vi "Main.vi"(11 "Module Admin":refnum<class "Delacor_lib_QMH_Cloneable Module Admin.lvclass">) -> ()   [LabVIEW 2024, in "Clon.lvlib"]
doc: "This template is based off of the Queued Message Handler design pattern and the Queued Message Handler project template that ships with LabVIEW.\n\nThe main difference is that the queue is private to this module and communication between modules is performed via Broadcast and Request events.\n\nRequest events are wrapped in public API methods and are handled in the Event Handling Loop (EHL) of this VI. Any module can register for Broadcast events sent by this module. The EHL generates messages based on user interface actions.\n\nThe Message Handling Loop (MHL) processes messages generated by the EHL, or by other messages. The messages are string values, so new messages can be added easily to the Message Cases case structure in the MHL. Each message cluster can also provide an optional value for Message Data, which is a variant that can be converted to whatever message-specific data is required.\n_____\nBased on DQMH Dev Tools: Project Template 7.1.0.1503."
uses:
  Clon.lvlib
  <vilib>/Delacor/Delacor QMH/Libraries/Cloneable Module Admin_class/Delacor_lib_QMH_Cloneable Module Admin.lvclass
  C:/Program Files (x86)/National Instruments/LabVIEW 2024/vi.lib/Delacor/Delacor QMH/Libraries/Module Admin_class/Delacor_lib_QMH_Module Admin.lvclass
  Module Data--cluster.ctl
  Do Something Argument--cluster.ctl
  <vilib>/Delacor/Delacor QMH/Libraries/Cloneable Module Admin_class/Delacor_lib_QMH_Cloneable Module Admin.lvclass/Delacor_lib_QMH_Cloneable Module Admin.ctl
  <vilib>/Delacor/Delacor QMH/Libraries/Message Queue_class/Delacor_lib_QMH_Message Queue.lvclass/Delacor_lib_QMH_Message Queue.ctl
  Do Something Else Argument--cluster.ctl
  Do Something Else and Wait for Reply Argument--cluster.ctl
  Do Something Else and Wait (Reply Payload)--cluster.ctl
  Stop Argument--cluster.ctl
  <vilib>/Delacor/Delacor QMH/Libraries/Module Admin_class/Delacor_lib_QMH_Module Admin.lvclass/Delacor_lib_QMH_Module Admin.ctl
  <vilib>/Utility/miscctls.llb/LVPointTypeDef.ctl
  <vilib>/Delacor/Delacor QMH/Libraries/Message Queue_class/Delacor_lib_QMH_Enqueue Message (Single).vi
  <vilib>/Delacor/Delacor QMH/Libraries/Cloneable Module Admin_class/Delacor_lib_QMH_Get Module ID.vi
  <vilib>/Delacor/Delacor QMH/Libraries/Module Admin_class/Delacor_lib_QMH_Get External Launch.vi
  <vilib>/Delacor/Delacor QMH/Libraries/Message Queue_class/Delacor_lib_QMH_Message Queue.lvclass
  Evento DEmo Argument--cluster.ctl
panel:
  out "error out":errorcluster
  out "X":dbl
  out "Status":string
  in  "Simulate EHL Error":bool
  in  "Simulate MHL Error":bool
  in  "Do Something Else <Replace Me>":bool
  in  "Do Something <Replace Me>":bool
  # "These controls have associated \"Value Changed\" events configured in the Event Structure on the diagram.\n\nReplace them (and reconfigure the Event Structure) with the controls you need for your application. \n\nOther processes communicate with this Module via its Public API (wrappers for its Request Events).\n\nThis Module communicates with other processes via its Broadcast Events.\nAny process that wants to receive these messages can register for this module's Broadcast events."
  # "This template is for the DQMH framework. See the block diagram for more information on how to use this template."
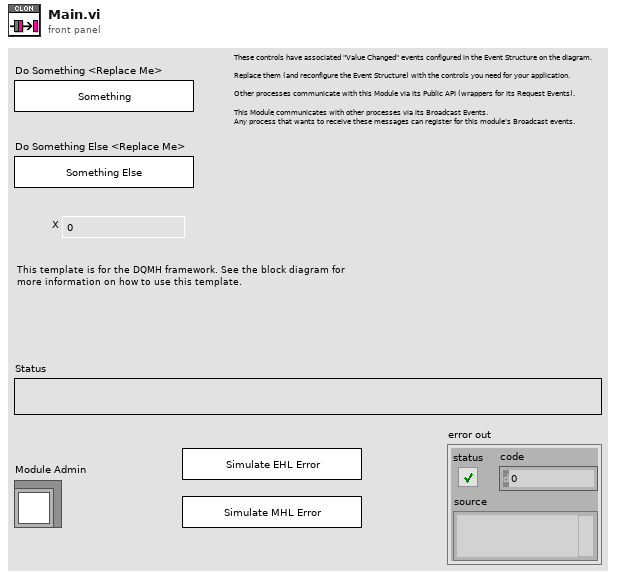
[diagram p1: front panel]
types:
  T1 = typedef "Clon.lvlib/Request Events--cluster.ctl" = cluster{"Stop Module":refnum<user-event>, "Do Something":refnum<user-event>, "Do Something Else":refnum<user-event>, "Do Something Else and Wait for Reply":refnum<user-event>, "Show Panel":refnum<user-event>, "Hide Panel":refnum<user-event>, "Show Diagram":refnum<user-event>, "Get Module Execution Status":refnum<user-event>, "Evento DEmo":refnum<user-event>}
  T2 = typedef "Clon.lvlib/Module Data--cluster.ctl" = cluster{"Status":string}
  T3 = typedef "Clon.lvlib/Do Something Argument--cluster.ctl" = cluster{"Module ID":i32, "Do Something Msg":string}
  T4 = typedef "Clon.lvlib/Do Something Else Argument--cluster.ctl" = cluster{"Module ID":i32, "Do Something Else Msg":string, "X":dbl}
  T5 = typedef "Clon.lvlib/Do Something Else and Wait for Reply Argument--cluster.ctl" = cluster{"Module ID":i32, "Do Something Else Msg":string, "X":dbl, "Wait Notifier":refnum<notifier>, "wait for reply":bool}
  T6 = enum32{"invalid lock state", "Not Locked", "Locked (No Password)", "Password-protected"}
  T7 = typedef "Clon.lvlib/Stop Argument--cluster.ctl" = cluster{"Module ID":i32, "Origin":string, "Exit via Stop Module Req?":bool, "Wait for Module to stop?":bool}
  T8 = typedef "Clon.lvlib/Evento DEmo Argument--cluster.ctl" = cluster{"Module ID":i32, "Numeric":dbl}
  T9 = typedef "LVPointTypeDef.ctl" = cluster{"Horizontal":i16, "Vertical":i16}
  T10 = enum32{"Invalid", "Standard", "Closed", "Hidden", "Minimized", "Maximized"}
  T11 = typedef "Clon.lvlib/Do Something Else and Wait (Reply Payload)--cluster.ctl" = cluster{"Value":dbl, "error":errorcluster, "Module ID":i32}
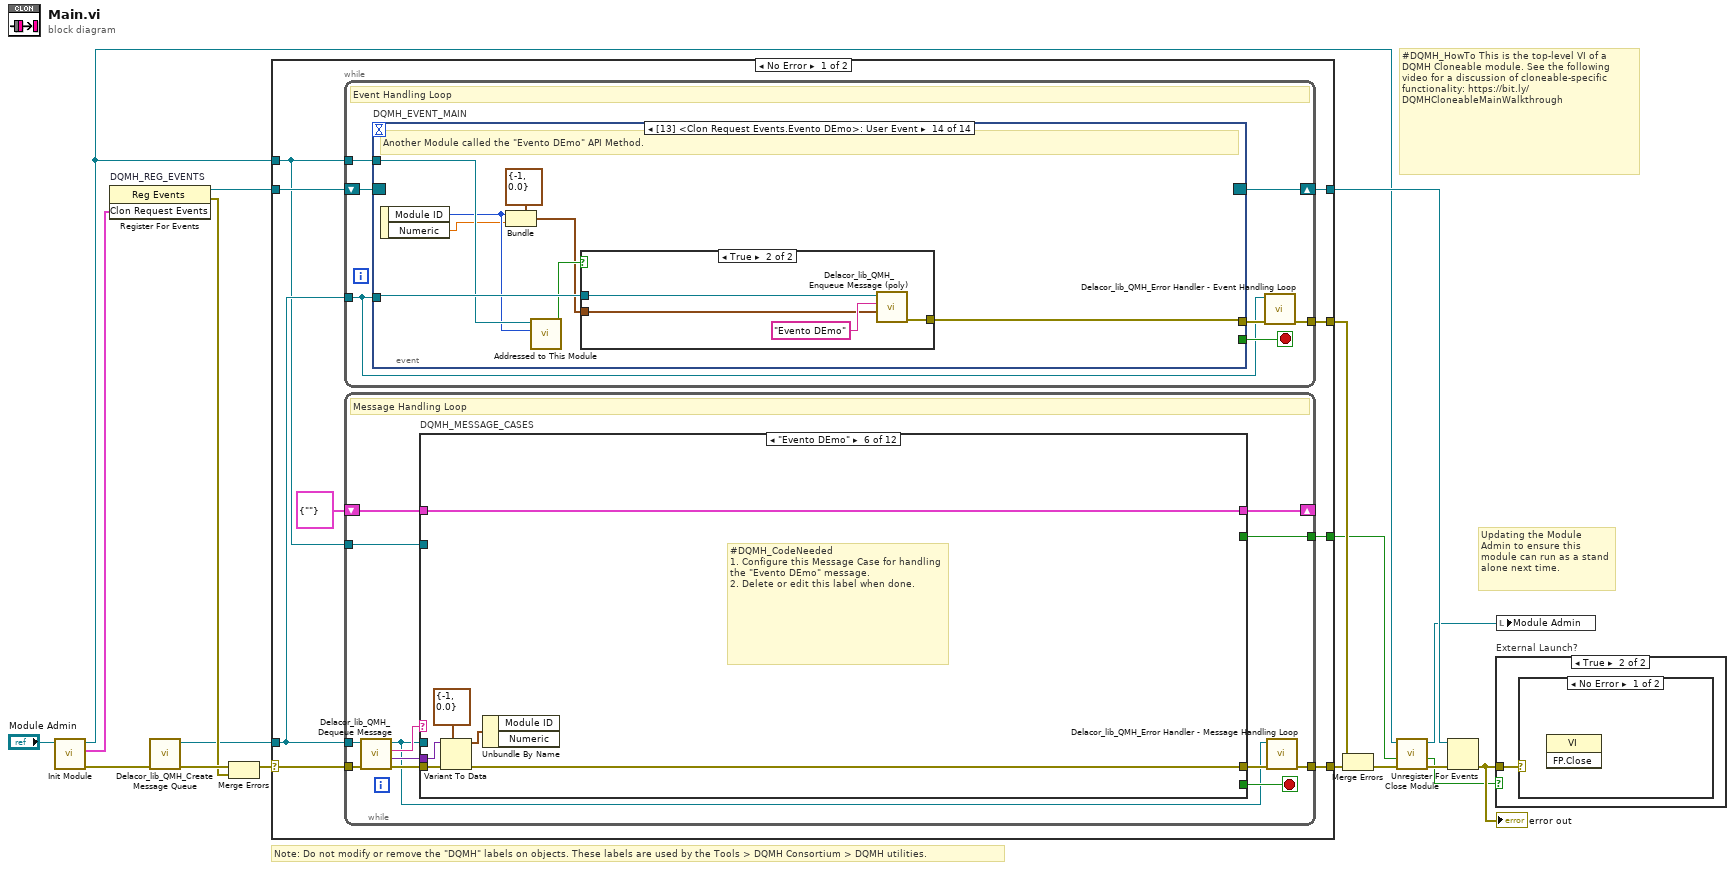
[diagram p0: block diagram]
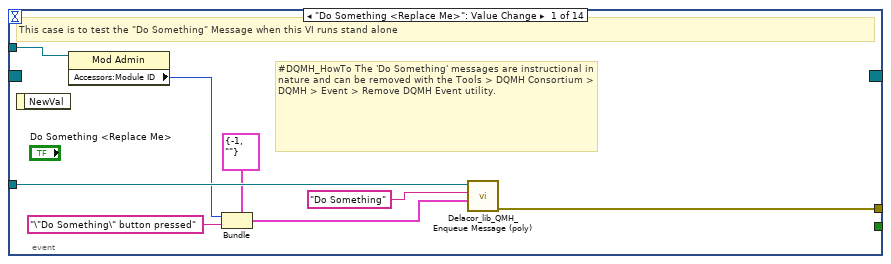
[diagram p2: hidden frame]
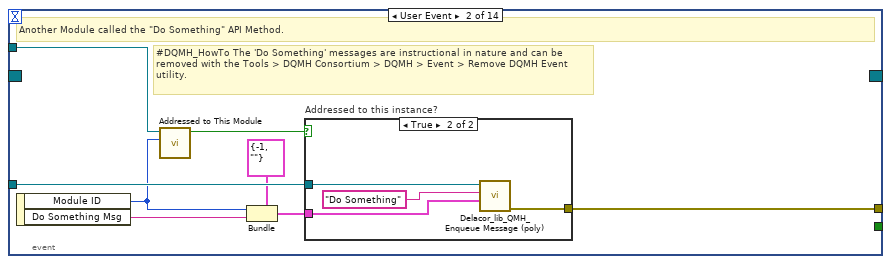
[diagram p3: hidden frame]
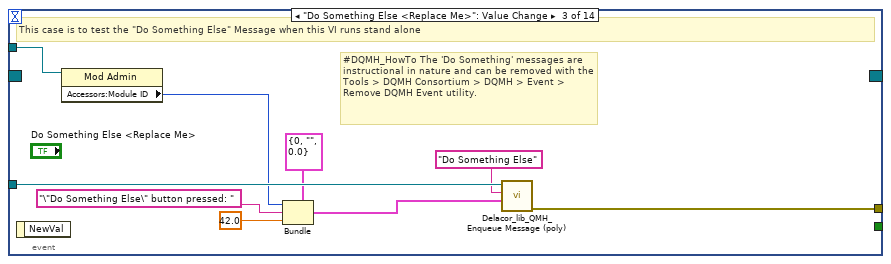
[diagram p5: hidden frame]
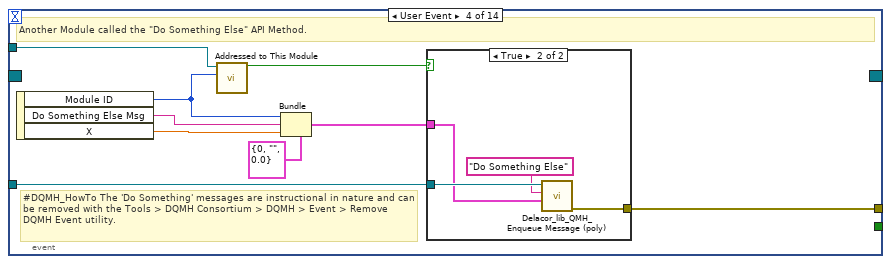
[diagram p6: hidden frame]
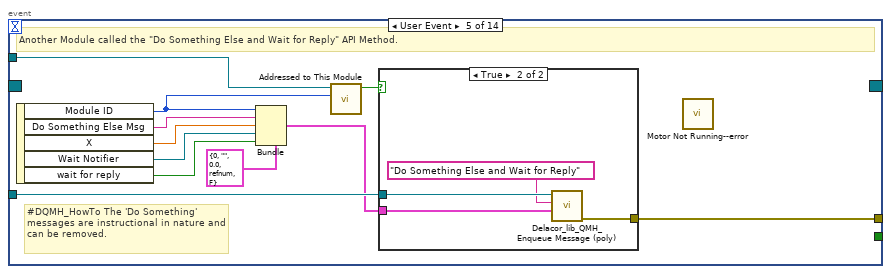
[diagram p8: hidden frame]
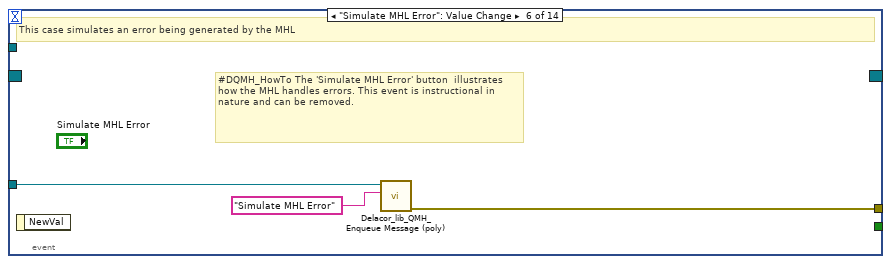
[diagram p10: hidden frame]
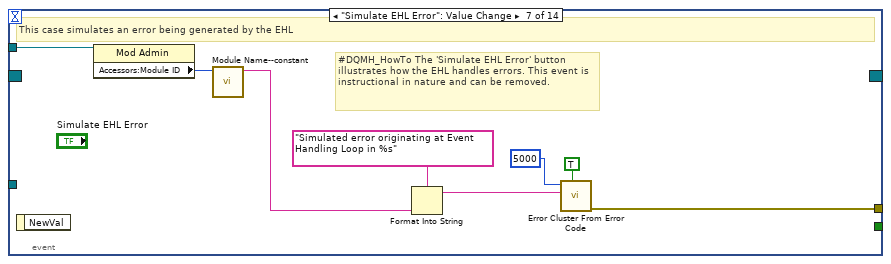
[diagram p11: hidden frame]
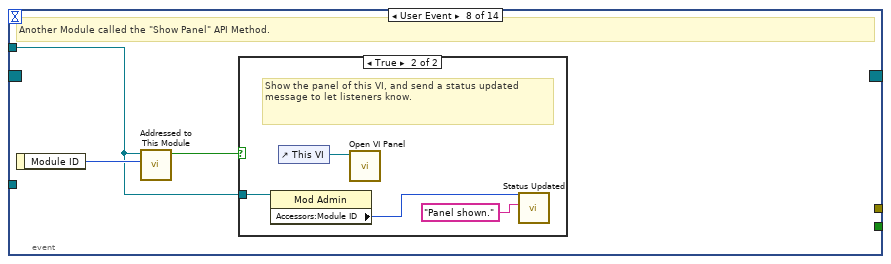
[diagram p12: hidden frame]
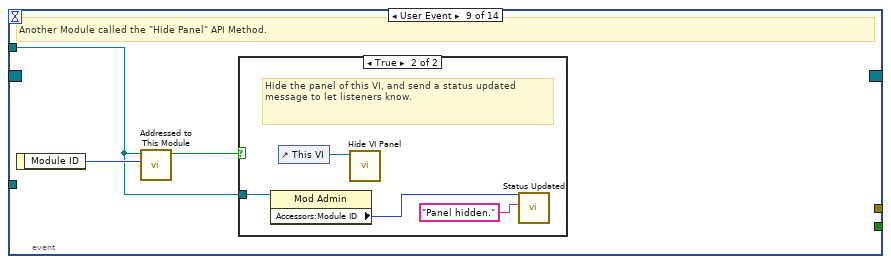
[diagram p14: hidden frame]
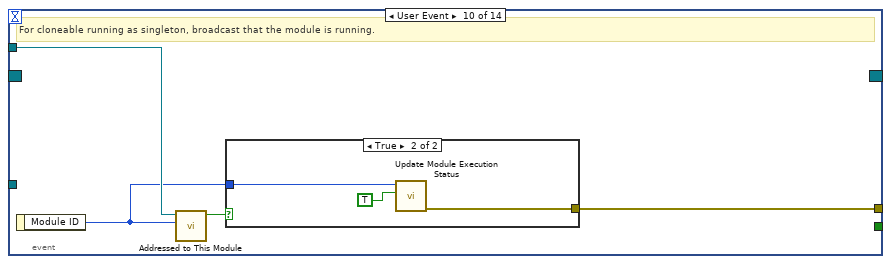
[diagram p16: hidden frame]
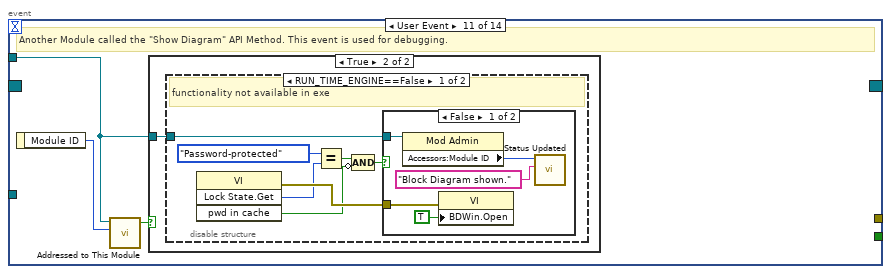
[diagram p18: hidden frame]
diagram:
  # "#DQMH_HowTo This is the top-level VI of a DQMH Cloneable module. See the following video for a discussion of cloneable-specific functionality: https://bit.ly/DQMHCloneableMainWalkthrough"
  # "Note: Do not modify or remove the \"DQMH\" labels on objects. These labels are used by the Tools > DQMH Consortium > DQMH utilities."
  # "Updating the Module Admin to ensure this module can run as a stand alone next time."
  n1 = call "Init Module.vi"("Cloneable Module Admin in"="Module Admin") -> ("error out"=w15:errorcluster, "Clon Request Events"=w7:T1, "Cloneable Module Admin out"=w4:refnum<class "Delacor_lib_QMH_Cloneable Module Admin.lvclass">)  [unwired: 8 in]
  n2 = register-events "DQMH_REG_EVENTS"(w7) -> (reference out=w8:refnum<event-registration>, error out=w10:errorcluster)  [unwired: 2 in]
  n3 = call <vilib>:"Delacor_lib_QMH_Create Message Queue.vi"("error in"=w15) -> ("error out"=w12:errorcluster, "Message Queue"=w6:refnum<class "Delacor_lib_QMH_Message Queue.lvclass">)  [unwired: 9 in]
  n4 = Merge Errors(w12, w10) -> (w11:errorcluster)
  n5 = case shown="No Error" w11 {
    selector: w11 -> [w25 w354]
    tunnel: [w27 w353] -> w16
    tunnel: [w24 w352] -> w9
    tunnel: w8 -> [w22 w352]
    tunnel: w6 -> [w21 w345]
    tunnel: [w26 _] -> w17
    tunnel: w4 -> [w20 w348]
    tunnel: [w19 _] -> w2
    frame No Error {
      n6 = while {
        tunnel: w21 -> [w28]
        shift-right: [w31] -> w24
        shift-left: w22 -> [w32]
        tunnel: [w33] -> w26
        tunnel: w20 -> [w29]
        stop <- w30 stop-if-true
        # "Event Handling Loop"
        n7 = event "DQMH_EVENT_MAIN" shown="[13] <Clon Request Events.Evento DEmo>: User Event" {
          selector: w32 -> [_ _ _ _ _ _ _ _ _ _ _ _ _ _]
          dyn-events: [_ _ _ _ _ _ _ _ _ _ _ _ _ _] -> w31
          timeout: _ -> [_ _ _ _ _ _ _ _ _ _ _ _ _ _]
          tunnel: [_ _ _ _ _ _ _ _ _ _ _ w143 _ _] -> w30
          tunnel: w28 -> [w41 w49 w62 w71 w86 w93 _ _ _ _ _ w146 w163 w183]
          tunnel: [w42 w50 w63 w72 w87 w94 w102 _ _ w120 _ w147 w166 w176] -> w34
          tunnel: w29 -> [w37 w47 w56 w69 w84 _ w101 w103 w110 w118 w124 w145 w164 w181]
          event "Do Something <Replace Me>": Value Change {
            # "#DQMH_HowTo The 'Do Something' messages are instructional in nature and can be removed with the Tools > DQMH Consortium > DQMH > Event > Remove DQMH Event utility."
            # "This case is to test the \"Do Something\" Message when this VI runs stand alone"
            n8 = event-data() -> ()  [unwired: 1 in, 1 out]
            n9 = property on="Property Node" class="Mod Admin"(reference=w37) -> ("Accessors:Module ID"=w36:i32)  [unwired: 1 in, 2 out]
            n10 = Bundle(cluster=T3 {"Module ID"=-1, "Do Something Msg"=""} ("Do Something Argument"), "Module ID"=w36, "Do Something Msg"="\"Do Something\" button pressed" ("\"Do Something\" button pressed")) -> (w39:T3)
            n11 = call-poly <vilib>:"Delacor_lib_QMH_Enqueue Message (poly).vi"("Message Data"=w39, "Message"="Do Something", "Message Queue in"=w41) -> ("error out"=w42:errorcluster)  [unwired: 7 in, 1 out]
          }
          event User Event {
            # "#DQMH_HowTo The 'Do Something' messages are instructional in nature and can be removed with the Tools > DQMH Consortium > DQMH > Event > Remove DQMH Event utility."
            # "Another Module called the \"Do Something\" API Method."
            n12 = event-data() -> ("Module ID"=w44:i32, "Do Something Msg"=w43:string)  [unwired: 1 in]
            n13 = call "Addressed to This Module.vi"("Module ID from Argument"=w44, "Module Admin"=w47) -> ("Addressed to this instance?"=w48:bool)  [unwired: 8 in, 1 out]
            n14 = Bundle(cluster=T3 {"Module ID"=-1, "Do Something Msg"=""} ("Do Something Argument"), "Module ID"=w44, "Do Something Msg"=w43) -> (w46:T3)
            n15 = case "Addressed to this instance?" shown="True" w48 {
              tunnel: w49 -> [_ w53]
              tunnel: [_ w54] -> w50
              tunnel: w46 -> [_ w51]
              frame False {
                # "Do nothing"
              }
              frame True {
                n16 = call-poly <vilib>:"Delacor_lib_QMH_Enqueue Message (poly).vi"("Message Data"=w51, "Message"="Do Something", "Message Queue in"=w53) -> ("error out"=w54:errorcluster)  [unwired: 7 in, 1 out]
              }
            }
          }
          event "Do Something Else <Replace Me>": Value Change {
            # "#DQMH_HowTo The 'Do Something' messages are instructional in nature and can be removed with the Tools > DQMH Consortium > DQMH > Event > Remove DQMH Event utility."
            # "This case is to test the \"Do Something Else\" Message when this VI runs stand alone"
            n17 = event-data() -> ()  [unwired: 1 in, 1 out]
            n18 = property on="Property Node" class="Mod Admin"(reference=w56) -> ("Accessors:Module ID"=w55:i32)  [unwired: 1 in, 2 out]
            n19 = Bundle(cluster=T4 {"Module ID"=0, "Do Something Else Msg"="", "X"=0.0} ("Do Something Else Argument"), "Module ID"=w55, "Do Something Else Msg"="\"Do Something Else\" button pressed: " ("\"Do Something Else\" button pressed"), "X"=42.0) -> (w59:T4)
            n20 = call-poly <vilib>:"Delacor_lib_QMH_Enqueue Message (poly).vi"("Message Data"=w59, "Message"="Do Something Else", "Message Queue in"=w62) -> ("error out"=w63:errorcluster)  [unwired: 7 in, 1 out]
          }
          event User Event {
            # "#DQMH_HowTo The 'Do Something' messages are instructional in nature and can be removed with the Tools > DQMH Consortium > DQMH > Event > Remove DQMH Event utility."
            # "Another Module called the \"Do Something Else\" API Method."
            n21 = event-data() -> ("Module ID"=w64:i32, "Do Something Else Msg"=w65:string, "X"=w67:dbl)  [unwired: 1 in]
            n22 = call "Addressed to This Module.vi"("Module ID from Argument"=w64, "Module Admin"=w69) -> ("Addressed to this instance?"=w70:bool)  [unwired: 8 in, 1 out]
            n23 = Bundle(cluster=T4 {"Module ID"=0, "Do Something Else Msg"="", "X"=0.0} ("Do Something Else Argument"), "Module ID"=w64, "Do Something Else Msg"=w65, "X"=w67) -> (w66:T4)
            n24 = case shown="True" w70 {
              tunnel: w71 -> [_ w75]
              tunnel: [_ w76] -> w72
              tunnel: w66 -> [_ w73]
              frame False {
              }
              frame True {
                n25 = call-poly <vilib>:"Delacor_lib_QMH_Enqueue Message (poly).vi"("Message Data"=w73, "Message"="Do Something Else", "Message Queue in"=w75) -> ("error out"=w76:errorcluster)  [unwired: 7 in, 1 out]
              }
            }
          }
          event User Event {
            # "#DQMH_HowTo The 'Do Something' messages are instructional in nature and can be removed."
            # "Another Module called the \"Do Something Else and Wait for Reply\" API Method."
            n26 = event-data() -> ("Module ID"=w82:i32, "Do Something Else Msg"=w80:string, "X"=w79:dbl, "Wait Notifier"=w78:refnum<notifier>, "wait for reply"=w77:bool)  [unwired: 1 in]
            n27 = Bundle(cluster=T5 {"Module ID"=0, "Do Something Else Msg"="", "X"=0.0, "Wait Notifier"=refnum, "wait for reply"=FALSE} ("Do Something Else and Wait for Reply Argument"), "Module ID"=w82, "Do Something Else Msg"=w80, "X"=w79, "Wait Notifier"=w78, "wait for reply"=w77) -> (w81:T5)
            n28 = call "Addressed to This Module.vi"("Module ID from Argument"=w82, "Module Admin"=w84) -> ("Addressed to this instance?"=w85:bool)  [unwired: 8 in, 1 out]
            n29 = case shown="True" w85 {
              tunnel: [_ w91] -> w87
              tunnel: w86 -> [_ w90]
              tunnel: w81 -> [_ w88]
              frame False {
              }
              frame True {
                n30 = call-poly <vilib>:"Delacor_lib_QMH_Enqueue Message (poly).vi"("Message Data"=w88, "Message"="Do Something Else and Wait for Reply", "Message Queue in"=w90) -> ("error out"=w91:errorcluster)  [unwired: 7 in, 1 out]
              }
            }
            n31 = call "Motor Not Running--error.vi"() -> ()  [unwired: 11 in, 1 out]
          }
          event "Simulate MHL Error": Value Change {
            # "#DQMH_HowTo The 'Simulate MHL Error' button  illustrates how the MHL handles errors. This event is instructional in nature and can be removed."
            # "This case simulates an error being generated by the MHL"
            n32 = event-data() -> ()  [unwired: 1 in, 1 out]
            n33 = call-poly <vilib>:"Delacor_lib_QMH_Enqueue Message (poly).vi"("Message"="Simulate MHL Error", "Message Queue in"=w93) -> ("error out"=w94:errorcluster)  [unwired: 8 in, 1 out]
          }
          event "Simulate EHL Error": Value Change {
            # "#DQMH_HowTo The 'Simulate EHL Error' button  illustrates how the EHL handles errors. This event is instructional in nature and can be removed."
            # "This case simulates an error being generated by the EHL"
            n34 = event-data() -> ()  [unwired: 1 in, 1 out]
            n35 = property on="Property Node" class="Mod Admin"(reference=w101) -> ("Accessors:Module ID"=w100:i32)  [unwired: 1 in, 2 out]
            n36 = call "Module Name--constant.vi"("Module ID"=w100) -> ("Module Name"=w95:string)  [unwired: 10 in]
            n37 = Format Into String(format string="Simulated error originating at Event Handling Loop in %s", w95) -> (resulting string=w98:string)  [unwired: 2 in, 1 out]
            n38 = call <vilib>:"Error Cluster From Error Code.vi"("show call chain? (False)"=TRUE, "error message (\"\")"=w98, "error code (0)"=5000) -> ("error out"=w102:errorcluster)  [unwired: 6 in]
          }
          event User Event {
            # "Another Module called the \"Show Panel\" API Method."
            n39 = event-data() -> ("Module ID"=w104:i32)  [unwired: 1 in]
            n40 = call "Addressed to This Module.vi"("Module ID from Argument"=w104, "Module Admin"=w103) -> ("Addressed to this instance?"=w105:bool)  [unwired: 8 in, 1 out]
            n41 = case shown="True" w105 {
              tunnel: w103 -> [_ w107]
              frame False {
              }
              frame True {
                # "Show the panel of this VI, and send a status updated message to let listeners know."
                n42 = property on="Property Node" class="Mod Admin"(reference=w107) -> ("Accessors:Module ID"=w106:i32)  [unwired: 1 in, 2 out]
                n43 = control-ref of="This VI"() -> (w109:refnum<vi>)
                n44 = call "Open VI Panel.vi"("VI"=w109) -> ()  [unwired: 10 in, 1 out]
                n45 = call "Status Updated.vi"("Status"="Panel shown." ("format string"), "Module ID"=w106) -> ()  [unwired: 9 in, 1 out]
              }
            }
          }
          event User Event {
            # "Another Module called the \"Hide Panel\" API Method."
            n46 = event-data() -> ("Module ID"=w111:i32)  [unwired: 1 in]
            n47 = call "Addressed to This Module.vi"("Module ID from Argument"=w111, "Module Admin"=w110) -> ("Addressed to this instance?"=w112:bool)  [unwired: 8 in, 1 out]
            n48 = case shown="True" w112 {
              tunnel: w110 -> [_ w114]
              frame False {
              }
              frame True {
                # "Hide the panel of this VI, and send a status updated message to let listeners know."
                n49 = property on="Property Node" class="Mod Admin"(reference=w114) -> ("Accessors:Module ID"=w113:i32)  [unwired: 1 in, 2 out]
                n50 = control-ref of="This VI"() -> (w116:refnum<vi>)
                n51 = call "Hide VI Panel.vi"("VI"=w116) -> ()  [unwired: 10 in, 1 out]
                n52 = call "Status Updated.vi"("Status"="Panel hidden." ("format string"), "Module ID"=w113) -> ()  [unwired: 9 in, 1 out]
              }
            }
          }
          event User Event {
            # "For cloneable running as singleton, broadcast that the module is running."
            n53 = event-data() -> ("Module ID"=w117:i32)  [unwired: 1 in]
            n54 = call "Addressed to This Module.vi"("Module ID from Argument"=w117, "Module Admin"=w118) -> ("Addressed to this instance?"=w119:bool)  [unwired: 8 in, 1 out]
            n55 = case shown="True" w119 {
              tunnel: [_ w123] -> w120
              tunnel: w117 -> [_ w122]
              frame False {
              }
              frame True {
                n56 = call "Update Module Execution Status.vi"("Running?"=TRUE, "Module ID"=w122) -> ("error out"=w123:errorcluster)  [unwired: 9 in]
              }
            }
          }
          event User Event {
            # "Another Module called the \"Show Diagram\" API Method. This event is used for debugging."
            n57 = event-data() -> ("Module ID"=w125:i32)  [unwired: 1 in]
            n58 = call "Addressed to This Module.vi"("Module ID from Argument"=w125, "Module Admin"=w124) -> ("Addressed to this instance?"=w126:bool)  [unwired: 8 in, 1 out]
            n59 = case shown="True" w126 {
              tunnel: w124 -> [_ w127]
              frame False {
              }
              frame True {
                n60 = disable-structure shown="RUN_TIME_ENGINE==False" {
                  disable-tunnel: w127 -> [w128 _]
                  frame condition #0 (active) {
                    # "functionality not available in exe"
                    n61 = invoke on="Invoke Node" class="VI" method="Lock State.Get"() -> (error out=w134:errorcluster, "Get Lock State"=w133:T6, "pwd in cache"=w130:bool)  [unwired: 4 in, 1 out]
                    n62 = Equal?(x=T6."Password-protected", y=w133) -> (x = y?=w131:bool)
                    n63 = Compound Arithmetic op=AND(w131, invert w130) -> (w129:bool)
                    n64 = case shown="False" w129 {
                      tunnel: w134 -> [w139 _]
                      tunnel: w128 -> [w136 _]
                      frame False {
                        n65 = property on="Property Node" class="Mod Admin"(reference=w136) -> ("Accessors:Module ID"=w135:i32)  [unwired: 1 in, 2 out]
                        n66 = property on="Property Node" class="VI"(error in=w139, "BDWin.Open"=TRUE ("Block Diagram Window:Open")) -> ()  [unwired: 1 in, 2 out]
                        n67 = call "Status Updated.vi"("Status"="Block Diagram shown." ("format string"), "Module ID"=w135) -> ()  [unwired: 9 in, 1 out]
                      }
                      frame True {
                        # "Password-protected VI, and the password is not in the cache. Do not show the diagram."
                      }
                    }
                  }
                  frame condition #1 {
                  }
                }
              }
            }
          }
          event User Event {
            # "Another Module called the \"Stop Module\" API Method  or the Message Handling Loop below."
            n68 = event-data() -> ("Module ID"=w141:i32, "Wait for Module to stop?"=w142:bool, "Origin"=w140:string)  [unwired: 1 in]
            n69 = call "Addressed to This Module.vi"("Module ID from Argument"=w141, "Module Admin"=w145) -> ("Addressed to this instance?"=w144:bool)  [unwired: 8 in, 1 out]
            n70 = case shown="True" w144 {
              tunnel: [_ w159] -> w147
              tunnel: w146 -> [_ w155]
              tunnel: [_ TRUE] -> w143
              tunnel: w142 -> [_ w150]
              tunnel: w141 -> [_ w152]
              tunnel: w140 -> [_ w148]
              frame False {
              }
              frame True {
                # "The event can get fired from the Exit message. The queue gets destroyed there. In this case, the Enqueue VI will return error 1. It is safe to ignore, because the module is already exiting."
                n71 = local write "Status"(w148) -> ()
                n72 = Bundle By Name(cluster=T7 {"Module ID"=-1, "Origin"="", "Exit via Stop Module Req?"=FALSE, "Wait for Module to stop?"=FALSE} ("Stop Argument"), "Module ID"=w152, "Exit via Stop Module Req?"=TRUE, "Wait for Module to stop?"=w150) -> (w149:T7)
                n73 = call-poly <vilib>:"Delacor_lib_QMH_Enqueue Message (poly).vi"("Priority Message? (F)"=TRUE, "Message Data"=w149, "Message"="Exit", "Message Queue in"=w155) -> ("error out"=w160:errorcluster)  [unwired: 6 in, 1 out]
                n74 = call <vilib>:"Clear Errors.vi"("error in (no error)"=w160, "specific error code to clear (0: all)"=1) -> ("error out"=w159:errorcluster)  [unwired: 4 in, 1 out]
              }
            }
          }
          event Panel Close? {
            w165 = TRUE  # Discard the event, the MHL is responsible for closing and stopping this VI.
            # "Hide the panel or send the 'Exit' message if the user clicks the 'X' on the module main VI panel."
            n75 = event-data() -> ()  [unwired: 1 in, 1 out]
            n76 = property on="Property Node" class="Mod Admin"(reference=w164) -> (reference out=w161:refnum<class "Delacor_lib_QMH_Cloneable Module Admin.lvclass">, "Accessors:External Launch"=w162:bool)  [unwired: 1 in, 1 out]
            n77 = case shown="True" w162 {
              tunnel: w163 -> [_ w174]
              tunnel: [_ w175] -> w166
              tunnel: w161 -> [w169 _]
              frame True {
                # "If externally launched, clicking the 'X' hides the panel, but doesn't close it."
                n78 = property on="Property Node" class="Mod Admin"(reference=w169) -> ("Accessors:Module ID"=w168:i32)  [unwired: 1 in, 2 out]
                n79 = call "Status Updated.vi"("Status"="Panel hidden." ("format string"), "Module ID"=w168) -> ("error out"=w167:errorcluster)  [unwired: 9 in]
                n80 = control-ref of="This VI"() -> (w171:refnum<vi>)
                n81 = call "Hide VI Panel.vi"("error in"=w167, "VI"=w171) -> ()  [unwired: 9 in, 1 out]
              }
              frame False {
                # "If run as a stand-alone VI, clicking the panel 'X' stops the VI."
                n82 = call-poly <vilib>:"Delacor_lib_QMH_Enqueue Message (poly).vi"("Priority Message? (F)"=TRUE, "Message"="Exit", "Message Queue in"=w174) -> ("error out"=w175:errorcluster)  [unwired: 7 in, 1 out]
              }
            }
            n83 = event-data ("Event Filter Node")("Discard?"=w165) -> ()  [unwired: 1 in, 1 out]
          }
          event User Event {
            # "Another Module called the \"Evento DEmo\" API Method."
            n84 = event-data() -> ("Module ID"=w178:i32, "Numeric"=w177:dbl)  [unwired: 1 in]
            n85 = Bundle(cluster=T8 {"Module ID"=-1, "Numeric"=0.0} ("Evento DEmo Argument"), "Module ID"=w178, "Numeric"=w177) -> (w179:T8)
            n86 = call "Addressed to This Module.vi"("Module ID from Argument"=w178, "Module Admin"=w181) -> ("Addressed to this instance?"=w182:bool)  [unwired: 8 in, 1 out]
            n87 = case shown="True" w182 {
              tunnel: w183 -> [_ w187]
              tunnel: w179 -> [_ w185]
              tunnel: [_ w184] -> w176
              frame False {
              }
              frame True {
                n88 = call-poly <vilib>:"Delacor_lib_QMH_Enqueue Message (poly).vi"("Message Data"=w185, "Message"="Evento DEmo", "Message Queue in"=w187) -> ("error out"=w184:errorcluster)  [unwired: 7 in, 1 out]
              }
            }
          }
        }
        n89 = call-dynamic "Delacor_lib_QMH_Error Handler - Event Handling Loop.vi"("error in"=w34, "Message Queue in"=w28) -> ("dup error in"=w33:errorcluster)  [unwired: 8 in, 1 out]
      }
      n90 = while {
        tunnel: w21 -> [w188]
        shift-right: [w195] -> _
        shift-left: T2 {"Status"=""} ("Data Cluster") -> [w196]
        tunnel: w25 -> [w199]
        tunnel: [w197] -> w27
        tunnel: w20 -> [w190]
        tunnel: [w189] -> w19
        stop <- w194 stop-if-true
        # "Message Handling Loop"
        n91 = call-dynamic "Delacor_lib_QMH_Dequeue Message.vi"("error in"=w199, "Message Queue in"=w188) -> ("error out"=w198:errorcluster, "Message Data"=w192:variant, "Message"=w193:string, "Message Queue out"=w191:refnum<class "Delacor_lib_QMH_Message Queue.lvclass">)  [unwired: 6 in]
        n92 = case "DQMH_MESSAGE_CASES" shown="\"Evento DEmo\"" w193 {
          selector: w193 -> [_ _ _ _ _ _ _ _ _ _ _ w334]
          tunnel: w191 -> [_ _ _ _ _ _ _ _ w289 _ w326 _]
          tunnel: w198 -> [w219 w223 w233 w244 w265 w281 w284 w286 w298 w315 w332 w343]
          tunnel: [w217 w223 w231 w243 w264 w279 w283 w286 w294 w314 w327 w344] -> w200
          tunnel: w196 -> [w210 w222 w230 w242 w245 w280 w282 w285 w293 w312 w325 w341]
          tunnel: [w209 w222 w230 w242 w245 w280 w282 w285 w293 w312 w325 w341] -> w195
          tunnel: [_ _ _ _ _ _ _ _ _ _ w324 _] -> w194
          tunnel: w192 -> [_ _ w229 w239 w259 w278 _ _ w292 _ w322 _]
          tunnel: w190 -> [w205 _ w225 w235 w250 _ _ _ w291 w310 w317 w340]
          tunnel: [_ _ _ _ _ _ _ _ _ _ w320 _] -> w189
          frame "Initialize" {
            w202 = "Initial Message" ("Initial Message")
            # "#DQMH_CodeNeeded - Initialize the appearance of the front panel."
            # "#DQMH_CodeNeeded - Initialize your state data here."
            # "Initialize - Any operation that needs to be done before the module can receive messages. Synchronize Caller Events.vi will inform Start Module.vi that the module has launched and is ready to receive messages. Module Did Init.vi will broadcast that the module initialized."
            n93 = call "Synchronize Caller Events.vi"("error in"=w219, "Module Admin"=w205) -> ("error out"=w218:errorcluster, "Module Admin out"=w204:refnum<class "Delacor_lib_QMH_Cloneable Module Admin.lvclass">)  [unwired: 8 in]
            n94 = property on="Property Node" class="Mod Admin"(reference=w204) -> ("Accessors:Module ID"=w201:i32, "Accessors:External Launch"=w206:bool)  [unwired: 1 in, 2 out]
            n95 = call "Module Name--constant.vi"("Module ID"=w201) -> ("Module Name"=w214:string)  [unwired: 10 in]
            n96 = property on="Property Node" class="VI"("Front Panel.Title"=w214) -> (reference out=w216:refnum<vi>, error out=w221:errorcluster)  [unwired: 2 in]
            n97 = Select(t=T10."Hidden" ("State"), s=w206, f=T10."Standard" ("State")) -> (s? t:f=w211:T10)
            n98 = invoke on="Invoke Node" class="VI" method="FP.Open"(reference=w216, error in=w221, "State"=w211) -> (reference out=w215:refnum<vi>, error out=w220:errorcluster)  [unwired: 2 in, 3 out]
            n99 = Bundle By Name(cluster=w210, "Status"=w202) -> (w209:T2)
            n100 = invoke on="Invoke Node" class="VI" method="FP.Center"(reference=w215, error in=w220) -> ()  [unwired: 1 in, 3 out]
            n101 = property on="Pane" class="Pane"("Origin"=T9 {"Horizontal"=0, "Vertical"=0}) -> ()  [unwired: 2 in, 2 out]
            n102 = call "Module Name--constant.vi"("Module ID"=w201) -> ("Module Name"=w207:string)  [unwired: 10 in]
            n103 = call "Module Did Init.vi"("error in"=w218, "Initialized?"=TRUE, "Origin"=w207, "Module ID"=w201) -> ("error out"=w217:errorcluster)  [unwired: 7 in]
            "Status" <- w202
          }
          frame "---Module Specific---" {
            # "Separator -- The following cases handle messages specific to this Module."
          }
          frame "Do Something" {
            # "#DQMH_HowTo The 'Do Something' messages are instructional in nature and can be removed with the Tools > DQMH Consortium > DQMH > Event > Remove DQMH Event utility."
            # "Do Something - Replace this message with functionality for your own application. Note that this message also fires the \"Did Something\" broadcast event."
            n104 = Variant To Data(error in=w233, type=T3 {"Module ID"=-1, "Do Something Msg"=""} ("Do Something Argument"), Variant=w229) -> (data=w228:T3, error out=w232:errorcluster)
            n105 = property on="Property Node" class="Mod Admin"(reference=w225) -> ("Accessors:Module ID"=w224:i32)  [unwired: 1 in, 2 out]
            n106 = Unbundle By Name(w228) -> ("Do Something Msg"=w226:string)
            n107 = call "Status Updated.vi"("Status"=w226, "Module ID"=w224) -> ()  [unwired: 9 in, 1 out]
            n108 = local write "Status"(w226) -> ()
            n109 = call "Did Something.vi"("error in"=w232, "Did Something Msg"=w226, "Module ID"=w224) -> ("error out"=w231:errorcluster)  [unwired: 8 in]
          }
          frame "Do Something Else" {
            # "#DQMH_HowTo The 'Do Something' messages are instructional in nature and can be removed with the Tools > DQMH Consortium > DQMH > Event > Remove DQMH Event utility."
            # "Do Something Else - Replace this message with functionality for your own application."
            n110 = Variant To Data(error in=w244, type=T4 {"Module ID"=0, "Do Something Else Msg"="", "X"=0.0} ("Do Something Else Argument"), Variant=w239) -> (data=w240:T4, error out=w243:errorcluster)
            n111 = Unbundle By Name(w240) -> ("Do Something Else Msg"=w238:string, "X"=w237:dbl)
            "X" <- w237
            n112 = property on="Property Node" class="Mod Admin"(reference=w235) -> ("Accessors:Module ID"=w234:i32)  [unwired: 1 in, 2 out]
            n113 = Format Into String(initial string=w238, w237) -> (resulting string=w236:string)  [unwired: 2 in, 1 out]
            n114 = call "Status Updated.vi"("Status"=w236, "Module ID"=w234) -> ()  [unwired: 9 in, 1 out]
            n115 = local write "Status"(w236) -> ()
          }
          frame "Do Something Else and Wait for Reply" {
            w252 = "X(%.2f)+Offset(%.2f)=%.2f"  # status message format string
            # "#DQMH_HowTo The 'Do Something' messages are instructional in nature and can be removed."
            # "Send back X with a random offset"
            # "Do Something Else and Wait for Reply - Replace this message with functionality for your own application. Note that this message must fire a notifier to let callers know it has finished execution, and it returns an error if the 'Value' is negative."
            n116 = property on="Property Node" class="Mod Admin"(reference=w250) -> ("Accessors:Module ID"=w247:i32)  [unwired: 1 in, 2 out]
            n117 = Variant To Data(error in=w265, type=T5 {"Module ID"=0, "Do Something Else Msg"="", "X"=0.0, "Wait Notifier"=refnum, "wait for reply"=FALSE} ("Do Something Else and Wait for Reply Argument"), Variant=w259) -> (data=w260:T5, error out=w263:errorcluster)
            n118 = Unbundle By Name(w260) -> ("Wait Notifier"=w257:refnum<notifier>, "Do Something Else Msg"=w258:string, "X"=w254:dbl, "wait for reply"=w248:bool)
            n119 = Random Number (0-1)() -> (number: 0 to 1=w253:dbl)
            n120 = Add(x=w253, y=w254) -> (x+y=w249:dbl)
            n121 = Less Than 0?(x=w249) -> (x < 0?=w246:bool)
            n122 = local write "X"(w254) -> ()
            n123 = case shown="True" w246 {
              tunnel: [_ w269] -> w262
              frame False {
              }
              frame True {
                n124 = call <vilib>:"Error Cluster From Error Code.vi"("show call chain? (False)"=TRUE, "error message (\"\")"="The 'Something Else and Wait for Reply' message generated a negative number, which is considered an error condition.", "error code (0)"=5000) -> ("error out"=w269:errorcluster)  [unwired: 6 in]
              }
            }
            n125 = Format Into String(format string=w252, initial string=w258, w254, w253, w249) -> (resulting string=w251:string)  [unwired: 1 in, 1 out]
            n126 = Bundle By Name(cluster=T11 {"Value"=0.0, "error"={"status"=FALSE, "code"=0, "source"=""}, "Module ID"=0} ("notification"), "error"=w262, "Value"=w249, "Module ID"=w247) -> (w255:T11)
            n127 = call "Status Updated.vi"("Status"=w251, "Module ID"=w247) -> ()  [unwired: 9 in, 1 out]
            n128 = local write "Status"(w251) -> ()
            n129 = case shown="False" w248 {
              tunnel: w257 -> [_ w273]
              tunnel: w255 -> [_ w272]
              frame False {
              }
              frame True {
                # "Simulate an operation that requires a wait."
                n130 = flat-sequence {
                  tunnel: w273 -> [w275]
                  tunnel: w272 -> [w274]
                  tunnel: w270 -> [_]
                  frame #0 {
                    n131 = Send Notification(notification=w274, notifier=w275) -> ()  [unwired: 1 in, 2 out]
                  }
                }
                n132 = Wait (ms)(milliseconds to wait=u32 1000) -> (millisecond timer value=w270:u32)
              }
            }
            n133 = Merge Errors(w263, w262) -> (w264:errorcluster)
          }
          frame "Evento DEmo" {
            # "#DQMH_CodeNeeded\n1. Configure this Message Case for handling the \"Evento DEmo\" message.\n2. Delete or edit this label when done."
            n134 = Variant To Data(error in=w281, type=T8 {"Module ID"=-1, "Numeric"=0.0} ("Evento DEmo Argument"), Variant=w278) -> (data=w276:T8, error out=w279:errorcluster)
            n135 = Unbundle By Name(w276) -> ()  [unwired: 2 out]
          }
          frame "---Copy This Frame---" {
            # "Duplicate this frame when creating new messages.  Change this comment in the duplicated frame to describe this message."
            n136 = Merge Errors(w284) -> (w283:errorcluster)
          }
          frame "---Exit and Error Handling---" {
            # "Separator - the following cases handle errors and exit messages."
          }
          frame "Error" {
            # "#DQMH_CodeRecommended - If the module is running in standalone mode (External Launch = FALSE), this code will pop up an error dialog and call the 'Exit' message if an error occurs. Add more fine-grained error management here."
            # "Error - Check the error message data and respond accordingly. This message is sent by the \"Error Handler\" VIs at the end of each loop in this application."
            n137 = property on="Property Node" class="Mod Admin"(reference=w291) -> ("Accessors:External Launch"=w290:bool, "Accessors:Module ID"=w288:i32)  [unwired: 1 in, 2 out]
            n138 = Variant To Data(error in=w298, type=errorcluster {"status"=FALSE, "code"=0, "source"=""} ("error constant"), Variant=w292) -> (data=w287:errorcluster, error out=w296:errorcluster)
            n139 = local write "error out"(w287) -> ()
            n140 = call "Error Reported.vi"("Error"=w287, "Module ID"=w288) -> ()  [unwired: 9 in, 1 out]
            n141 = case shown="False" w290 {
              tunnel: [w303 _] -> w295
              tunnel: w289 -> [w301 _]
              tunnel: w287 -> [w302 _]
              frame False {
                n142 = disable-structure shown="Default" {
                  disable-tunnel: w302 -> [w304 _]
                  frame condition #0 (active) {
                    # "If the module is running standalone, then pop up an error dialog and call the \"Exit\" message."
                    n143 = call <vilib>:"Simple Error Handler.vi"("error in (no error)"=w304) -> ()  [unwired: 4 in, 5 out]
                  }
                  frame condition #1 {
                    # "To prevent the Simple Error Handler VI from being loaded (e.g. when deploying to a Real-Time target), add the Conditional Disable Symbol \"DQMH_Disable_SEH\" to your project and set it to TRUE."
                  }
                }
                n144 = call-poly <vilib>:"Delacor_lib_QMH_Enqueue Message (poly).vi"("Priority Message? (F)"=TRUE, "Message"="Exit", "Message Queue in"=w301) -> ("error out"=w303:errorcluster)  [unwired: 7 in, 1 out]
              }
              frame True {
                # "If the module was launched externally, calling the Error Reported broadcast VI is the only action performed by the \"Error\" message. The module's caller can then process the error appropriately."
              }
            }
            n145 = Merge Errors(w296, w295) -> (w294:errorcluster)
          }
          frame "Simulate MHL Error" {
            # "#DQMH_HowTo The 'Simulate MHL Error' button  illustrates how the MHL handles errors. This event is instructional in nature and can be removed."
            # "Simulate an error occurring at the MHL"
            n146 = property on="Property Node" class="Mod Admin"(reference=w310) -> ("Accessors:Module ID"=w311:i32)  [unwired: 1 in, 2 out]
            n147 = call "Module Name--constant.vi"("Module ID"=w311) -> ("Module Name"=w306:string)  [unwired: 10 in]
            n148 = Format Into String(format string="Simulated error originating at Message Handling Loop in %s", w306) -> (resulting string=w307:string)  [unwired: 2 in, 1 out]
            n149 = call <vilib>:"Error Cluster From Error Code.vi"("show call chain? (False)"=TRUE, "error message (\"\")"=w307, "error code (0)"=5001) -> ("error out"=w313:errorcluster)  [unwired: 6 in]
            n150 = Merge Errors(w315, w313) -> (w314:errorcluster)
          }
          frame "Exit" {
            w323 = 91  # 91: not all Exit messages will have an argument
            w324 = TRUE  # Stop the VI
            # "Release the message queue reference"
            # "#DQMH_CodeNeeded - Add any required cleanup code here."
            # "Exit - Exit the application."
            n151 = Variant To Data(error in=w332, type=T7 {"Module ID"=-1, "Origin"="", "Exit via Stop Module Req?"=FALSE, "Wait for Module to stop?"=FALSE} ("Stop Argument"), Variant=w322) -> (data=w319:T7, error out=w328:errorcluster)
            n152 = call <vilib>:"Clear Errors.vi"("error in (no error)"=w328, "specific error code to clear (0: all)"=w323) -> ("error out"=w331:errorcluster)  [unwired: 4 in, 1 out]
            n153 = property on="Property Node" class="Mod Admin"(reference=w317) -> ("Accessors:Module ID"=w316:i32)  [unwired: 1 in, 2 out]
            n154 = control-ref of="This VI"() -> (w318:refnum<vi>)
            n155 = call-dynamic "Delacor_lib_QMH_Release Message Queue.vi"("error in"=w331, "Message Queue"=w326) -> ("error out"=w330:errorcluster)  [unwired: 9 in]
            n156 = call "Handle Exit.vi"("Stop Argument"=w319, "Module Admin in"=w317, "VI reference"=w318) -> ("error out"=w329:errorcluster, "Wait for Stop?"=w320:bool)  [unwired: 7 in]
            n157 = Merge Errors(w330, w329) -> (w327:errorcluster)
            n158 = call "Error Reported.vi"("Error"=w327, "Module ID"=w316) -> ()  [unwired: 9 in, 1 out]
          }
          frame Default {
            # "'Default' case only runs if there is a message that isn't defined in any of the other cases.  Output a programming error."
            n159 = property on="Property Node" class="Mod Admin"(reference=w340) -> ("Accessors:Module ID"=w339:i32)  [unwired: 1 in, 2 out]
            n160 = call "Module Name--constant.vi"("Module ID"=w339) -> ("Module Name"=w333:string)  [unwired: 10 in]
            n161 = Format Into String(format string="The invalid message string \"%s\" was received in the Message Handling Loop for module \"%s\".", w334, w333) -> (resulting string=w336:string)  [unwired: 2 in, 1 out]
            n162 = call <vilib>:"Error Cluster From Error Code.vi"("show call chain? (False)"=TRUE, "error message (\"\")"=w336, "error code (0)"=1) -> ("error out"=w342:errorcluster)  [unwired: 6 in]
            n163 = Merge Errors(w343, w342) -> (w344:errorcluster)
          }
        }
        n164 = call-dynamic "Delacor_lib_QMH_Error Handler - Message Handling Loop.vi"("error in"=w200, "Message Queue in"=w191) -> ("dup error in"=w197:errorcluster)  [unwired: 8 in, 1 out]
      }
    }
    frame Error {
      n165 = call "Synchronize Caller Events.vi"("Module Admin"=w348) -> ("Module Admin out"=w347:refnum<class "Delacor_lib_QMH_Cloneable Module Admin.lvclass">)  [unwired: 9 in, 1 out]
      n166 = property on="Property Node" class="Mod Admin"(reference=w347) -> ("Accessors:Module ID"=w346:i32)  [unwired: 1 in, 2 out]
      n167 = call-dynamic "Delacor_lib_QMH_Release Message Queue.vi"("error in"=w354, "Message Queue"=w345) -> ("error out"=w353:errorcluster)  [unwired: 9 in]
      n168 = call "Module Name--constant.vi"("Module ID"=w346) -> ("Module Name"=w351:string)  [unwired: 10 in]
      n169 = Format Into String(format string="An error occurred during initialization. %s is no longer running.", w351) -> (resulting string=w349:string)  [unwired: 2 in, 1 out]
      n170 = call "Error Reported.vi"("Additional Information"=w349, "Error"=w353, "Module ID"=w346) -> ()  [unwired: 8 in, 1 out]
    }
  }
  n171 = Merge Errors(w17, w16) -> (w18:errorcluster)
  n172 = call "Close Module.vi"("error in"=w18, "Wait for stop?"=w2, "Module Admin in"=w4) -> ("error out"=w14:errorcluster, "External Launch"=w1:bool, "Module Admin out"=w3:refnum<class "Delacor_lib_QMH_Cloneable Module Admin.lvclass">)  [unwired: 6 in]
  n173 = Unregister For Events(event registration refnum=w9, error in=w14) -> (error out=w13:errorcluster)
  "error out" <- w13
  n174 = case "External Launch?" shown="True" w1 {
    tunnel: w13 -> [_ w355]
    frame False {
    }
    frame True {
      n175 = case shown="No Error" w355 {
        frame No Error {
          n176 = invoke class="VI" method="FP.Close"() -> ()  [unwired: 3 in, 3 out]
        }
        frame Error {
          n177 = disable-structure shown="Default" {
            frame condition #0 (active) {
              n178 = invoke class="VI" method="FP.Open"("Activate"=TRUE ("Activate?")) -> ()  [unwired: 4 in, 5 out]
            }
            frame condition #1 {
              # "Don't show panel on error if running inside a built EXE."
            }
          }
        }
      }
    }
  }
  n179 = local write "Module Admin"(w3) -> ()
